vi "test Timestamp.vi"(11 "Test Case In":refnum<class "Test PCANBasic.lvclass">) -> (0 "error out":errorcluster, 3 "Test Case Out":refnum<class "Test PCANBasic.lvclass">)   [LabVIEW 2020, in "Test PCANBasic.lvclass"]
uses:
  Test PCANBasic.lvclass
  source/PCANBasic.lvlib
  Global PCAN Channel.vi
  Global PCAN Baudrate.vi
  <vilib>/Astemes/LUnit/Test Case.lvclass
  source/Read Event/Read Event.lvclass
panel:
  out "abs diff":dbl
  out "Time Stamp":timestamp format="%<%x %.3X>T"
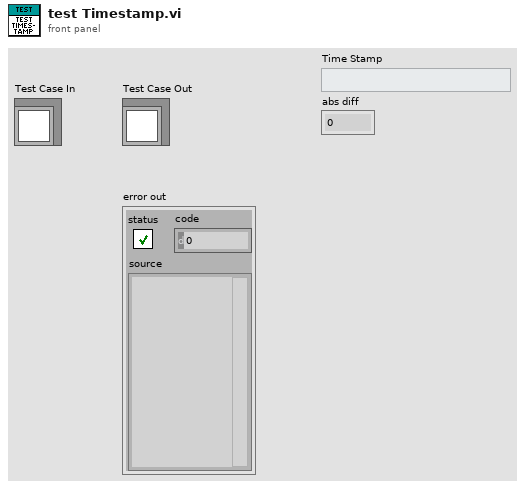
[diagram p1: front panel]
types:
  T1 = cluster{"ID":u32, "MSGTYPE":cluster{"Type":u8, "Extended":bool, "Echo":bool}, "LEN":u8, "DATA":cluster{"0":u8, "1":u8, "2":u8, "3":u8, "4":u8, "5":u8, "6":u8, "7":u8}}
  T2 = cluster{"0":u8, "1":u8, "2":u8, "3":u8, "4":u8, "5":u8, "6":u8, "7":u8}
  T3 = typedef "PCANBasic.lvlib/PCAN Baud.ctl" = u16
  T4 = typedef "PCANBasic.lvlib/TPCANHandle.ctl" = u16
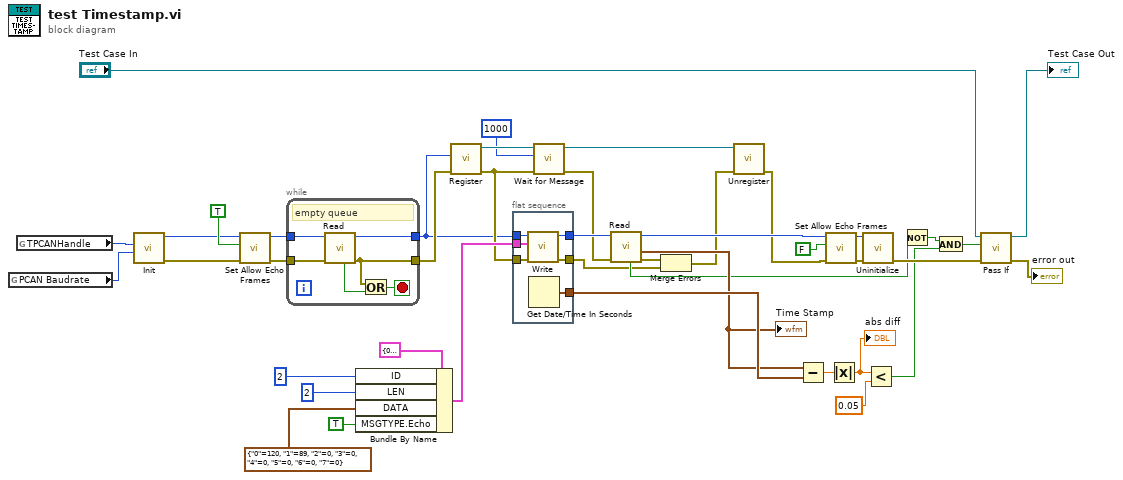
[diagram p0: block diagram]
diagram:
  n1 = global read "Global PCAN Baudrate.vi" "PCAN Baudrate"() -> (w39:T3)
  n2 = global read "Global PCAN Channel.vi" "TPCANHandle"() -> (w38:T4)
  n3 = call "Init.vi"("Baudrate"=w39, "Channel"=w38) -> ("error out"=w13:errorcluster, "TPCANHandle out"=w11:T4)  [unwired: 7 in, 1 out]
  n4 = call "Set Allow Echo Frames.vi"("error in"=w13, "Enable"=TRUE, "TPCANHandle in"=w11) -> ("error out"=w31:errorcluster, "TPCANHandle out"=w30:T4)  [unwired: 6 in, 1 out]
  n5 = while {
    tunnel: w31 -> [w48]
    tunnel: [w44] -> w12
    tunnel: w30 -> [w47]
    tunnel: [w46] -> w5
    stop <- w45 stop-if-true
    # "empty queue"
    n6 = call "Read.vi"("error in"=w48, "TPCANHandle in"=w47) -> ("error out"=w44:errorcluster, "TPCANHandle out"=w46:T4, "Receive Queue empty"=w43:bool)  [unwired: 4 in, 3 out]
    n7 = Or(x=w44, y=w43) -> (x .or. y?=w45:bool)
  }
  n8 = Bundle By Name(cluster=T1 {"ID"=0, "MSGTYPE"={"Type"=0, "Extended"=FALSE, "Echo"=FALSE}, "LEN"=0, "DATA"={"0"=0, "1"=0, "2"=0, "3"=0, "4"=0, "5"=0, "6"=0, "7"=0}} ("PCAN Message"), "ID"=u32 2, "LEN"=u8 2, "DATA"=T2 {"0"=120, "1"=89, "2"=0, "3"=0, "4"=0, "5"=0, "6"=0, "7"=0}, "MSGTYPE.Echo"=TRUE) -> (w33:T1)
  n9 = call "Register.vi"("error in"=w12, "TPCANHandle"=w5) -> ("error out"=w10:errorcluster, "Read Event out"=w15:refnum<class "Read Event.lvclass">)  [unwired: 8 in]
  n10 = flat-sequence {
    tunnel: [w54] -> w1
    tunnel: w33 -> [w53]
    tunnel: [w50] -> _
    tunnel: w5 -> [w52]
    tunnel: [w51] -> w23
    tunnel: w10 -> [w50]
    tunnel: [w49] -> w4
    frame #0 {
      n11 = call "Write.vi"("error in"=w50, "PCAN Message"=w53, "TPCANHandle in"=w52) -> ("error out"=w54:errorcluster, "TPCANHandle out"=w49:T4)  [unwired: 6 in, 1 out]
      n12 = Get Date/Time In Seconds() -> (seconds since 1Jan1904=w51:timestamp)
    }
  }
  n13 = call "Wait for Message.vi"("error in"=w10, "Timeout"=1000, "Read Event in"=w15) -> ("error out"=w3:errorcluster, "Read Event out"=w9:refnum<class "Read Event.lvclass">)  [unwired: 6 in, 1 out]
  n14 = call "Read.vi"("error in"=w3, "TPCANHandle in"=w4) -> ("error out"=w8:errorcluster, "Time Stamp"=w19:timestamp, "TPCANHandle out"=w26:T4, "Receive Queue empty"=w16:bool)  [unwired: 4 in, 2 out]
  "Time Stamp" <- w19
  n15 = Merge Errors(w8, w1) -> (w2:errorcluster)
  n16 = call "Unregister.vi"("error in"=w2, "Read Event in"=w9) -> ("error out"=w7:errorcluster)  [unwired: 8 in, 1 out]
  n17 = Subtract(x=w19, y=w23) -> (x-y=w22:dbl)
  n18 = call "Set Allow Echo Frames.vi"("error in"=w7, "Enable"=FALSE, "TPCANHandle in"=w26) -> ("error out"=w27:errorcluster, "TPCANHandle out"=w25:T4)  [unwired: 6 in, 1 out]
  n19 = Absolute Value(x=w22) -> (abs(x)=w6:dbl)
  "abs diff" <- w6
  n20 = call "Uninitialize.vi"("error in"=w27, "TPCANHandle in"=w25) -> ("error out"=w28:errorcluster)  [unwired: 8 in, 1 out]
  n21 = Less?(x=w6, y=0.05) -> (x < y?=w20:bool)
  n22 = Not(x=w16) -> (.not. x?=w17:bool)
  n23 = And(x=w17, y=w20) -> (x .and. y?=w18:bool)
  n24 = call <vilib>:"Pass If.vi"("error in (no error)"=w28, "Pass?"=w18, "LUnit Test Case In"="Test Case In") -> ("error out"=→"error out":errorcluster, "LUnit Test Case Out"=→"Test Case Out":refnum<class "Test PCANBasic.lvclass">)  [unwired: 7 in]
